vi "Generate Unexpexted Channel Error.vi"(8 "error in (no error)":errorcluster, 11 "Unexpected Channel Names":string[](array[string])) -> (0 "error out":errorcluster)   [LabVIEW 2020, in "Error Provider API.lvlib"]
uses:
  <vilib>/NI VeriStand/Error Provider API/Error Provider API.lvlib
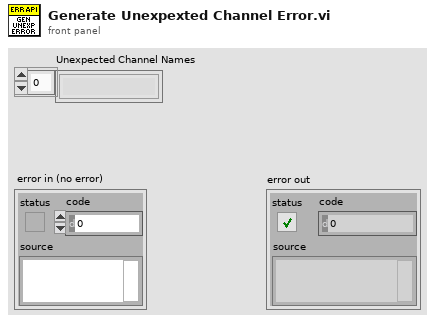
[diagram p1: front panel]
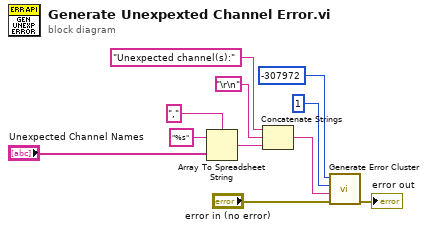
[diagram p0: block diagram]
diagram:
  n1 = Array To Spreadsheet String(delimiter (Tab)=",", array="Unexpected Channel Names", 3:"%s" ("format string")) -> (spreadsheet string=w8:string)
  n2 = Concatenate Strings("Unexpected channel(s):" ("source"), "\r\n", w8) -> (w3:string)
  n3 = call <vilib>:"Generate Error Cluster.vi"("error in (no error)"="error in (no error)", "Additional Message"=w3, "CallChainLvl (-1 => No call chain)"=1, "Code"=-307972) -> ("error out"=→"error out":errorcluster)  [unwired: 7 in]
